vi "CtrlRef.vi"() -> ()   [LabVIEW 2020]
panel:
  in  "Input":string caption="输入"
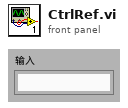
[diagram p1: front panel]
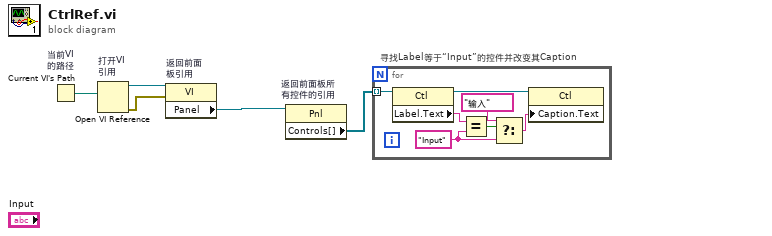
[diagram p0: block diagram]
diagram:
  # "寻找Label等于“Input”的控件并改变其Caption"
  n1 = Current VI's Path "当前VI\n的路径"() -> (path=w5:path)
  n2 = Open VI Reference "打开VI\n引用"(vi path=w5) -> (vi reference=w4:refnum<vi>, error out=w3:errorcluster)  [unwired: 1 in, 4 out]
  n3 = property on="返回前面\n板引用" class="VI"(reference=w4, error in=w3) -> ("Panel"=w2:refnum<vi>)  [unwired: 2 out]
  n4 = property on="返回前面板所\n有控件的引用" class="Pnl"(reference=w2) -> ("Controls[]"=w1:refnum<vi>[])  [unwired: 1 in, 2 out]
  n5 = for {
    tunnel: w1 -> [w12] mode=indexing
    w6 = "Input" ("y")
    n6 = property class="Ctl"(reference=w12) -> (reference out=w9:refnum<vi>, "Label.Text"=w11:string)  [unwired: 1 in, 1 out]
    n7 = Equal?(x=w11, y=w6) -> (x = y?=w10:bool)
    n8 = Select(t="输入" ("y"), s=w10, f=w6) -> (s? t:f=w8:string)
    n9 = property class="Ctl"(reference=w9, "Caption.Text"=w8) -> ()  [unwired: 1 in, 2 out]
  }
